vi "LauncherAngleTalon.vi"() -> ()   [LabVIEW 2013]
uses:
  State_Machine_Enum.ctl
  RefnameEnum.ctl
  Sally_Dashboard_2014/DBNameEnum.ctl
  Robot Global Data.vi
panel:
  in  "Start at bottom?":bool=TRUE
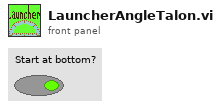
[diagram p1: front panel]
types:
  T1 = typedef "State_Machine_Enum.ctl" = enum16{"Idle", "Start", "Do", "Stop", "Init"}
  T2 = typedef "RefnameEnum.ctl" = enum16{"FireLauncher", "Climber", "Shield", "TankDrive", "DriveEncoderL", "DriveEncoderR", "LauncherMotorRPM", "LauncherEncoderAnalog", "LauncherEncoderRPM", "ShooterLS", "DriveAlignLSLeft", "DriveAlignLSRight", "ClimbingLS", "LauncherEncoderAngle", "LauncherMotorAngle", "Gamepad1", "Gamepad2", "Compressor", "ClimbWeightSol3", "ClimbWeightSol4"}
  T3 = typedef "DBNameEnum.ctl" = enum16{"AutoInstructions", "DriveLoopTime", "DriveAlignLSLeft", "DriveAlignLSRight", "Use2DriveAlign", "ClimbLS", "LauncherAngleMatches", "FrameworkVersion", "sLauncherAngle", "LauncherTargetAngle", "sLauncherRPM", "LauncherTargetRPM", "sDriveDistance", "LauncherMotorValue", "PullbackTol", "FireTol", "LauncherRPMTol", "LauncherAngleTol", "InitialWait", "WaitBetweenLaunch", "AnglePresets", "RPMPresets", "UseAngleEncoder", "UseLauncherEncoder", "UseLauncherPID", "QSWaitBeforeFire", "QSWaitBeforeRetract", "AngleForwardValue", "AngleBackwardValue", "UseClusterArray", "BackupAuto", "ReverseDriveIndicate", "HalfSpeedFactor"}
  T4 = typedef "LoopDisable.ctl" = cluster{"Climb.vi":bool, "LauncherAngle.vi":bool, "Launcher.vi":bool, "ArmControl.vi":bool, "WinchMotor.vi":bool, "ReadDriveEncoder.vi":bool}
  T5 = typedef "WPI_EncoderDevRef.ctl" = cluster{"DevStatus":errorcluster, "EncoderIndex":T6, "CounterIndex":T7, "DistancePerCount":dbl, "Decoding Type":T8}
  T6 = typedef "FPGA_EncoderIdx.ctl" = enum8{"Enc 0", "Enc 1", "Enc 2", "Enc 3", "Invalid"}
  T7 = typedef "FPGA_CounterCtrSystemIndex.ctl" = enum8{"Ctr 0", "Ctr 1", "Ctr 2", "Ctr 3", "Ctr 4", "Ctr 5", "Ctr 6", "Ctr 7", "Invalid"}
  T8 = typedef "WPI_EncoderType.ctl" = enum16{"1x", "2x", "4x"}
  T9 = typedef "WPI_DigitalInputDevRef.ctl" = cluster{"DevStatus":errorcluster, "DIO Channel":T10, "Digital Module":T11}
  T10 = typedef "FPGA_DIOChannel.ctl" = enum8{"DIO 1", "DIO 2", "DIO 3", "DIO 4", "DIO 5", "DIO 6", "DIO 7", "DIO 8", "DIO 9", "DIO 10", "DIO 11", "DIO 12", "DIO 13", "DIO 14", "Invalid"}
  T11 = typedef "FPGA_TypedefDigitalModule.ctl" = enum16{"Digital Module 1", "Digital Module 2"}
  T12 = typedef "WPI_MotorControlDeviceRef.ctl" = cluster{"DeviceStatus":errorcluster, "Type":enum16{"PWM", "CAN"}, "PWM":cluster{"Digital Module":T11, "PWM Channel":T13, "DeadBand":T14}, "CAN":cluster{"Device Number":u8, "Control Mode":T15, "Semaphore":T16, "Max Vout":dbl}, "Invert":bool, "TransformRef":T17, "InvTransformRef":T17}
  T13 = typedef "FPGA_DIOPWMChannel.ctl" = enum8{"PWM 1", "PWM 2", "PWM 3", "PWM 4", "PWM 5", "PWM 6", "PWM 7", "PWM 8", "PWM 9", "PWM 10", "Invalid"}
  T14 = typedef "WPI_PWMDeadband.ctl" = cluster{"Name":string, "maxPositivePwm":i32, "minPositivePwm":i32, "centerPwm":i32, "maxNegativePwm":i32, "minNegativePwm":i32, "angularRange":u16}
  T15 = typedef "WPI_CANJaguar_ControlMode.ctl" = enum8{"Percent VBus", "Current", "Speed", "Position", "Voltage"}
  T16 = typedef "Semaphore RefNum" = refnum<k1>
  T17 = typedef "WPI_PWMTransform_ConPane.ctl" = refnum<vi>
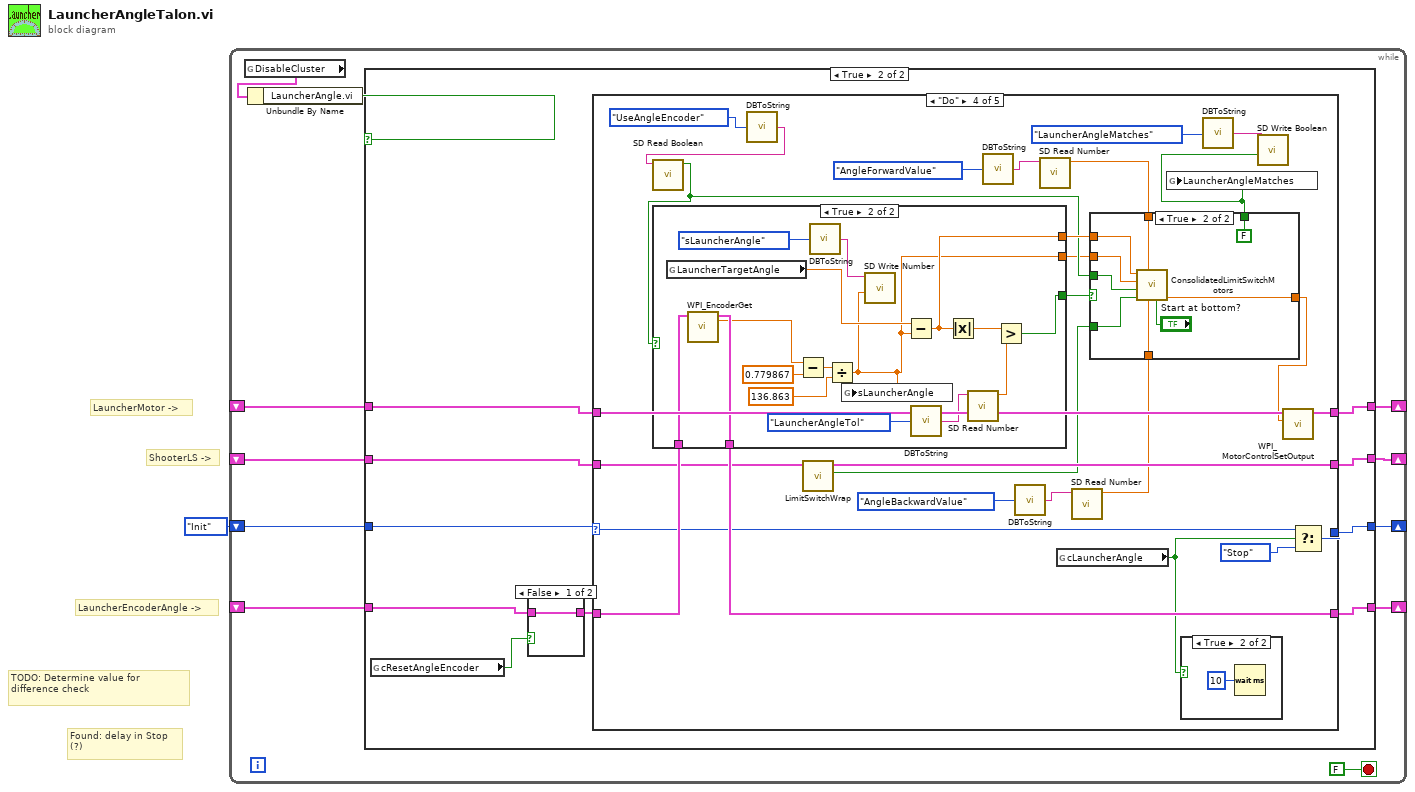
[diagram p0: block diagram]
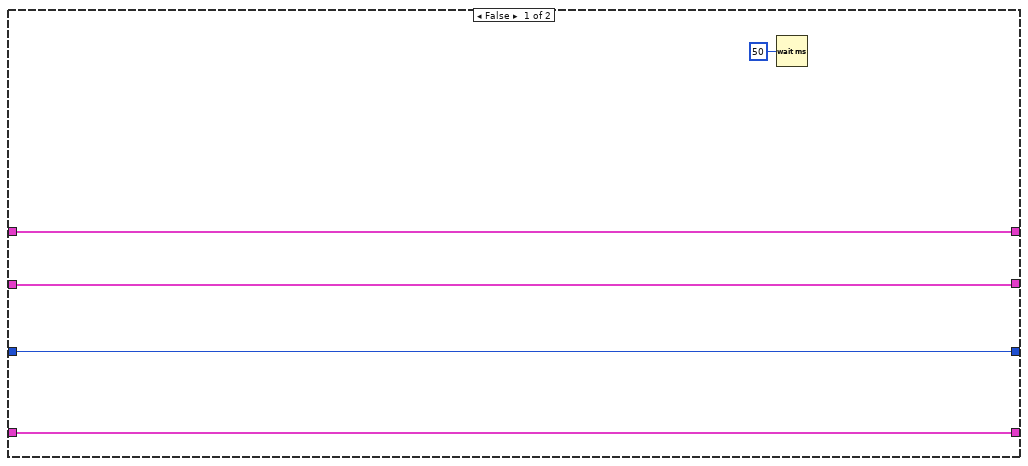
[diagram p2: hidden frame]
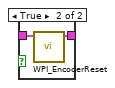
[diagram p3: hidden frame]
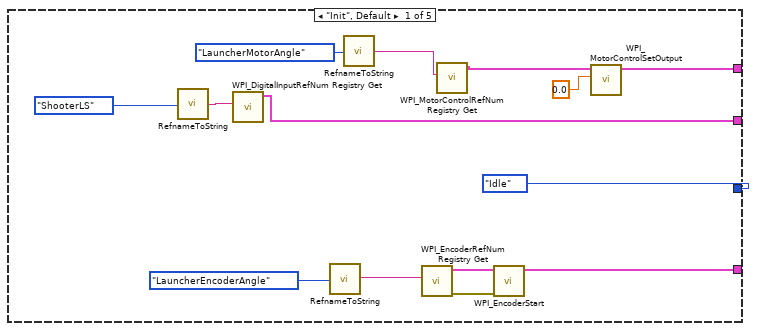
[diagram p4: hidden frame]
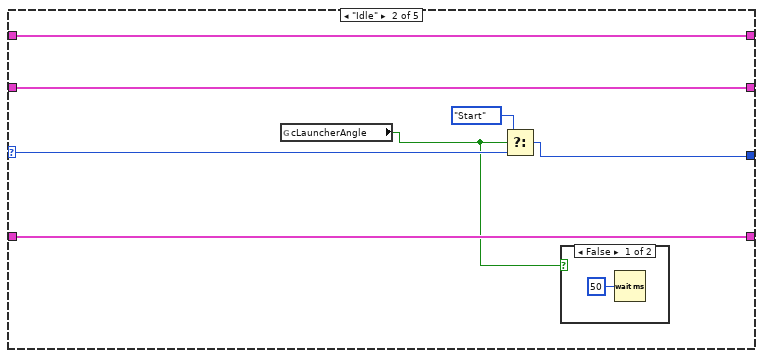
[diagram p5: hidden frame]
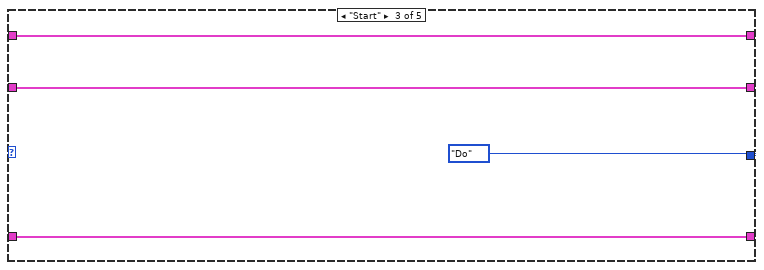
[diagram p7: hidden frame]
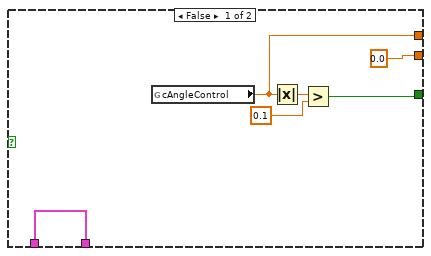
[diagram p8: hidden frame]
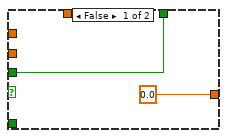
[diagram p10: hidden frame]
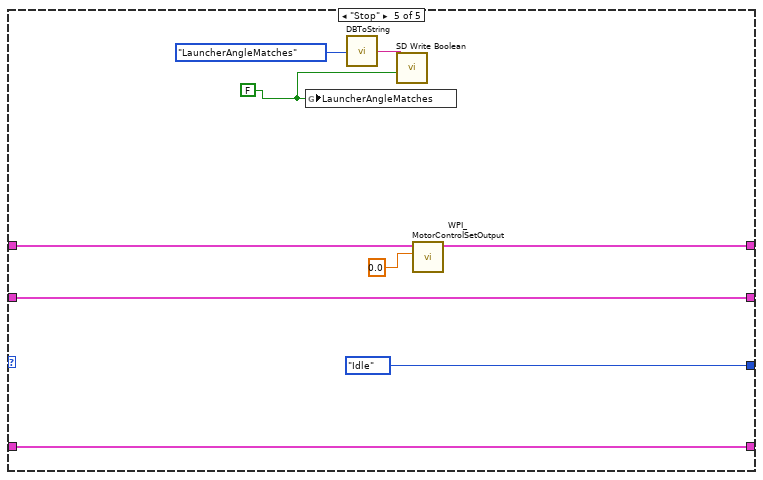
[diagram p11: hidden frame]
diagram:
  # "ShooterLS ->"
  # "Found: delay in Stop \n(?)"
  # "TODO: Determine value for difference check"
  # "LauncherEncoderAngle ->"
  # "LauncherMotor ->"
  n1 = while {
    shift-right: [w10] -> _
    shift-left: State_Machine_Enum."Init" ("State") -> [w11]
    shift-right: [w9] -> _
    shift-left: _ -> [w8]
    shift-right: [w4] -> _
    shift-left: _ -> [w3]
    shift-right: [w6] -> _
    shift-left: _ -> [w7]
    stop <- FALSE stop-if-true
    n2 = global read "Robot Global Data.vi" "DisableCluster"() -> (w5:T4)
    n3 = Unbundle By Name(w5) -> ("LauncherAngle.vi"=w2:bool)
    n4 = case shown="True" w2 {
      tunnel: w11 -> [w16 w27]
      tunnel: [w16 w26] -> w10
      tunnel: [w15 w25] -> w9
      tunnel: w8 -> [w15 w20]
      tunnel: w7 -> [w17 w24]
      tunnel: [w17 w23] -> w6
      tunnel: [w13 w22] -> w4
      tunnel: w3 -> [w13 w21]
      frame False {
        n5 = Wait (ms)(milliseconds to wait=u32 50) -> ()  [unwired: 1 out]
      }
      frame True {
        n6 = global read "Robot Global Data.vi" "cResetAngleEncoder"() -> (w18:bool)
        n7 = case shown="False" w18 {
          tunnel: w20 -> [w28 w30]
          tunnel: [w28 w29] -> w19
          frame False {
          }
          frame True {
            n8 = call <vilib>:"WPI_EncoderReset.vi"("EncoderDevRef"=w30) -> ("EncoderDevRef"=w29:T5)  [unwired: 9 in, 1 out]
          }
        }
        n9 = case shown="\"Do\"" w27 {
          selector: w27 -> [_ w49 _ w80 _]
          tunnel: [State_Machine_Enum."Idle" ("State") w50 State_Machine_Enum."Do" ("State") w79 State_Machine_Enum."Idle" ("State")] -> w26
          tunnel: [w42 w47 w55 w81 w126] -> w25
          tunnel: w19 -> [_ w47 w55 w82 w126]
          tunnel: w24 -> [_ w48 w54 w72 w125]
          tunnel: [w40 w48 w54 w71 w125] -> w23
          tunnel: [w39 w45 w53 w74 w123] -> w22
          tunnel: w21 -> [_ w45 w53 w75 w124]
          frame "Init", Default {
            n10 = call "RefnameToString.vi"("Enum"=RefnameEnum."ShooterLS") -> ("Refname"=w33:string)
            n11 = call <vilib>:"WPI_DigitalInputRefNum Registry Get.vi"("refnum name"=w33) -> ("DigitalInputDevRef"=w40:T9)  [unwired: 9 in, 1 out]
            n12 = call "RefnameToString.vi"("Enum"=RefnameEnum."LauncherEncoderAngle") -> ("Refname"=w31:string)
            n13 = call "RefnameToString.vi"("Enum"=RefnameEnum."LauncherMotorAngle") -> ("Refname"=w35:string)
            n14 = call <vilib>:"WPI_EncoderRefNum Registry Get.vi"("refnum name"=w31) -> ("error out"=w41:errorcluster, "EncoderDevRef"=w43:T5)  [unwired: 9 in]
            n15 = call <vilib>:"WPI_MotorControlRefNum Registry Get.vi"("refnum name"=w35) -> ("MotorControlDevRef"=w37:T12)  [unwired: 9 in, 1 out]
            n16 = call <vilib>:"WPI_EncoderStart.vi"("error in (no error)"=w41, "EncoderDevRef"=w43) -> ("EncoderDevRef"=w42:T5)  [unwired: 8 in, 1 out]
            n17 = call <vilib>:"WPI_MotorControlSetOutput.vi"("Output"=0.0, "MotorControlDevRef"=w37) -> ("MotorControlDevRef"=w39:T12)  [unwired: 7 in, 2 out]
          }
          frame "Idle" {
            n18 = global read "Robot Global Data.vi" "cLauncherAngle"() -> (w46:bool)
            n19 = Select(t=State_Machine_Enum."Start" ("State"), s=w46, f=w49) -> (s? t:f=w50:T1)
            n20 = case shown="False" w46 {
              frame False {
                n21 = Wait (ms)(milliseconds to wait=u32 50) -> ()  [unwired: 1 out]
              }
              frame True {
              }
            }
          }
          frame "Start" {
          }
          frame "Do" {
            n22 = call "DBToString.vi"("Enum"=DBNameEnum."UseAngleEncoder") -> ("Refname"=w63:string)
            n23 = call <vilib>:"SD Read Boolean.vi"("Name"=w63) -> ("Boolean"=w68:bool)  [unwired: 8 in, 2 out]
            n24 = case shown="True" w68 {
              tunnel: w82 -> [w85 w105]
              tunnel: [w85 w104] -> w81
              tunnel: [w86 w102] -> w78
              tunnel: [w87 w101] -> w77
              tunnel: [0.0 w96] -> w67
              frame False {
                n25 = global read "Robot Global Data.vi" "cAngleControl"() -> (w86:dbl)
                n26 = Absolute Value(x=w86) -> (abs(x)=w89:dbl)
                n27 = Greater?(x=w89, y=0.1) -> (0:w87:bool)
              }
              frame True {
                n28 = global read "Robot Global Data.vi" "LauncherTargetAngle"() -> (w97:dbl)
                n29 = call <vilib>:"WPI_EncoderGet.vi"("EncoderDevRef"=w105) -> ("Distance"=w90:dbl, "EncoderDevRef"=w104:T5)  [unwired: 5 in, 4 out]
                n30 = Subtract(x=w90, y=0.779867) -> (x-y=w100:dbl)
                n31 = call "DBToString.vi"("Enum"=DBNameEnum."sLauncherAngle") -> ("Refname"=w91:string)
                n32 = Divide(x=w100, y=136.863) -> (x/y=w96:dbl)
                n33 = global write "Robot Global Data.vi" "sLauncherAngle"(w96) -> ()
                n34 = call <vilib>:"SD Write Number.vi"("Numeric"=w96, "Name"=w91) -> ()  [unwired: 8 in, 2 out]
                n35 = Subtract(x=w97, y=w96) -> (x-y=w102:dbl)
                n36 = call "DBToString.vi"("Enum"=DBNameEnum."LauncherAngleTol") -> ("Refname"=w93:string)
                n37 = Absolute Value(x=w102) -> (abs(x)=w103:dbl)
                n38 = call <vilib>:"SD Read Number.vi"("Name"=w93) -> ("Numeric"=w95:dbl)  [unwired: 8 in, 2 out]
                n39 = Greater?(x=w103, y=w95) -> (0:w101:bool)
              }
            }
            n40 = call "LimitSwitchWrap.vi"("DigitalInputDevRef"=w72) -> ("Triggered"=w70:bool, "DigitalInputDevRef 2"=w71:T9)  [unwired: 9 in]
            n41 = call "DBToString.vi"("Enum"=DBNameEnum."AngleForwardValue") -> ("Refname"=w61:string)
            n42 = call "DBToString.vi"("Enum"=DBNameEnum."AngleBackwardValue") -> ("Refname"=w58:string)
            n43 = call <vilib>:"SD Read Number.vi"("Name"=w61) -> ("Numeric"=w60:dbl)  [unwired: 8 in, 2 out]
            n44 = global read "Robot Global Data.vi" "cLauncherAngle"() -> (w76:bool)
            n45 = call <vilib>:"SD Read Number.vi"("Name"=w58) -> ("Numeric"=w57:dbl)  [unwired: 8 in, 2 out]
            n46 = case shown="True" w77 {
              tunnel: w78 -> [_ w113]
              tunnel: [0.0 ("New Output") w117] -> w73
              tunnel: w70 -> [_ w116]
              tunnel: w57 -> [_ w115]
              tunnel: w60 -> [_ w114]
              tunnel: [w107 FALSE] -> w69
              tunnel: w68 -> [w107 w109]
              tunnel: w67 -> [_ w110]
              frame False {
              }
              frame True {
                n47 = call "ConsolidatedLimitSwitchMotors.vi"("Start at bottom?"="Start at bottom?", "BackwardValue"=w115, "ForwardValue"=w114, "CurrentLSValue"=w116, "UsingEncoder?"=w109, "AngleEncoderValue"=w110, "CurrentInput"=w113) -> ("New Output"=w117:dbl)  [unwired: 4 in]
              }
            }
            n48 = global write "Robot Global Data.vi" "LauncherAngleMatches"(w69) -> ()
            n49 = case shown="True" w76 {
              frame False {
              }
              frame True {
                n50 = Wait (ms)(milliseconds to wait=u32 10) -> ()  [unwired: 1 out]
              }
            }
            n51 = call "DBToString.vi"("Enum"=DBNameEnum."LauncherAngleMatches") -> ("Refname"=w65:string)
            n52 = call <vilib>:"SD Write Boolean.vi"("Boolean"=w69, "Name"=w65) -> ()  [unwired: 8 in, 2 out]
            n53 = call <vilib>:"WPI_MotorControlSetOutput.vi"("Output"=w73, "MotorControlDevRef"=w75) -> ("MotorControlDevRef"=w74:T12)  [unwired: 7 in, 2 out]
            n54 = Select(t=w80, s=w76, f=State_Machine_Enum."Stop" ("State")) -> (s? t:f=w79:T1)
          }
          frame "Stop" {
            w120 = FALSE
            n55 = global write "Robot Global Data.vi" "LauncherAngleMatches"(w120) -> ()
            n56 = call "DBToString.vi"("Enum"=DBNameEnum."LauncherAngleMatches") -> ("Refname"=w119:string)
            n57 = call <vilib>:"SD Write Boolean.vi"("Boolean"=w120, "Name"=w119) -> ()  [unwired: 8 in, 2 out]
            n58 = call <vilib>:"WPI_MotorControlSetOutput.vi"("Output"=0.0, "MotorControlDevRef"=w124) -> ("MotorControlDevRef"=w123:T12)  [unwired: 7 in, 2 out]
          }
        }
      }
    }
  }
